vi "Parsing Equations for Linear Optimization.vi"(10 "Variables":string, 11 "Equation":string) -> (0 "error out":errorcluster, 1 "Symbol output":string, 2 "left side":dbl, 3 "Vector":dbl[](array[numeric]), 4 "After symbol":string, 5 "Before symbol":string)   [LabVIEW 2023]
doc: "Parse equation for linear optimization."
uses:
  <vilib>/Utility/error.llb/Trim Whitespace One-Sided.vi
  <vilib>/gmath/NI_Gmath.lvlib
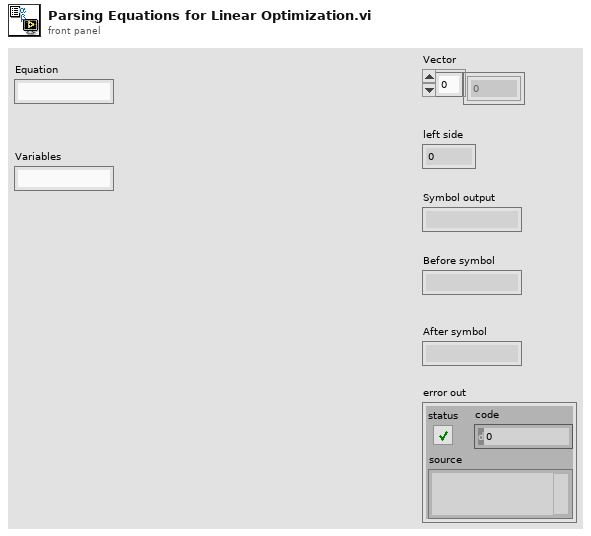
[diagram p1: front panel]
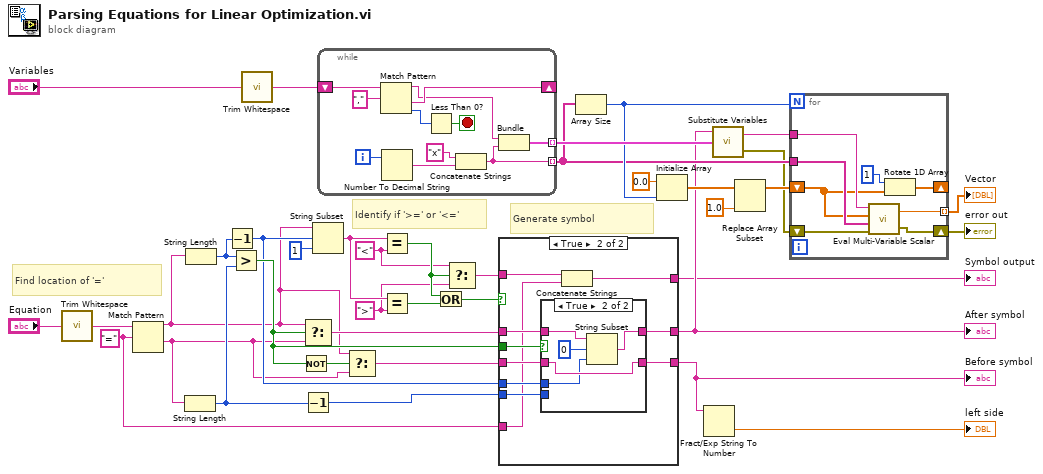
[diagram p0: block diagram]
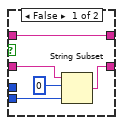
[diagram p3: hidden frame]
diagram:
  w5 = ">" ("y")
  w6 = "<" ("y")
  w9 = "=" ("symbol")
  # "Generate symbol"
  # "Identify if '>=' or '<='"
  # "Find location of '='"
  n1 = call <vilib>:"Trim Whitespace.vi"("string"="Equation") -> ("trimmed string"=w37:string)  [unwired: 1 in]
  n2 = Match Pattern(string=w37, regular expression=w9) -> (before substring=w2:string, after substring=w1:string)  [unwired: 1 in, 2 out]
  n3 = String Length(string=w1) -> (length=w13:i32)
  n4 = String Length(string=w2) -> (length=w15:i32)
  n5 = Decrement(x=w15) -> (x-1=w12:i32)
  n6 = Greater?(x=w15, y=w13) -> (0:w14:bool)
  n7 = call <vilib>:"Trim Whitespace.vi"("string"="Variables") -> ("trimmed string"=w35:string)  [unwired: 1 in]
  n8 = Not(x=w14) -> (.not. x?=w19:bool)
  n9 = Select(t=w2, s=w14, f=w1) -> (s? t:f=w16:string)
  n10 = Decrement(x=w13) -> (x-1=w18:i32)
  n11 = String Subset(string=w2, offset (0)=w12, length (rest)=1 ("length (rest)")) -> (substring=w22:string)
  n12 = while {
    shift-right: [w46] -> _
    shift-left: w35 -> [w45]
    tunnel: [w43] -> w34 mode=indexing
    tunnel: [w40] -> w26 mode=indexing
    i -> [w44]
    stop <- w47 stop-if-true
    n13 = Match Pattern(string=w45, regular expression=",") -> (before substring=w42:string, after substring=w46:string, offset past match=w48:i32)  [unwired: 1 in, 1 out]
    n14 = Number To Decimal String(number=w44) -> (decimal integer string=w41:string)  [unwired: 1 in]
    n15 = Less Than 0?(x=w48) -> (x < 0?=w47:bool)
    n16 = Concatenate Strings("x" ("string"), w41) -> (w40:string)
    n17 = Bundle("trimmed string"=w42, w40) -> (w43:cluster{"trimmed string":string, string})  [unwired: 1 in]
  }
  n18 = Select(t=w2, s=w19, f=w1) -> (s? t:f=w17:string)
  n19 = Equal?(x=w22, y=w6) -> (x = y?=w7:bool)
  n20 = Equal?(x=w22, y=w5) -> (x = y?=w23:bool)
  n21 = Or(x=w7, y=w23) -> (x .or. y?=w21:bool)
  n22 = Select(t=w6, s=w7, f=w5) -> (s? t:f=w4:string)
  n23 = case shown="True" w21 {
    tunnel: w16 -> [w52 w58]
    tunnel: w18 -> [_ w62]
    tunnel: [w52 w57] -> w20
    tunnel: w17 -> [w51 w61]
    tunnel: [w51 w60] -> w11
    tunnel: w14 -> [_ w59]
    tunnel: w12 -> [_ w56]
    tunnel: [w50 w54] -> w8
    tunnel: w9 -> [w50 w53]
    tunnel: w4 -> [_ w55]
    frame False {
    }
    frame True {
      n24 = case shown="True" w59 {
        tunnel: w62 -> [w66 _]
        tunnel: w61 -> [w65 w69]
        tunnel: [w64 w69] -> w60
        tunnel: w58 -> [w63 w71]
        tunnel: [w63 w70] -> w57
        tunnel: w56 -> [_ w68]
        frame False {
          n25 = String Subset(string=w65, offset (0)=0, length (rest)=w66) -> (substring=w64:string)
        }
        frame True {
          n26 = String Subset(string=w71, offset (0)=0, length (rest)=w68) -> (substring=w70:string)
        }
      }
      n27 = Concatenate Strings(w55, w53) -> (w54:string)
    }
  }
  "Before symbol" <- w11
  "Symbol output" <- w8
  "After symbol" <- w20
  n28 = Array Size(array=w26) -> (size(s)=w32:i32)
  n29 = Initialize Array(0.0 ("element"), w32) -> (w30:dbl[])
  n30 = Fract/Exp String To Number(string=w11) -> (number=→"left side":dbl)  [unwired: 3 in, 1 out]
  n31 = call <vilib>:"Substitute Variables.vi"("Substitution Rules"=w34, "original formula"=w20) -> ("error out"=w3:errorcluster, "formula after substitution"=w33:string)  [unwired: 1 in]
  n32 = Replace Array Subset(array=w30, new element=1.0 ("new element/subarray")) -> (w28:dbl[])  [unwired: 1 in]
  n33 = for {
    N: w32 -> [_]
    tunnel: w33 -> [w80]
    tunnel: [w79] -> w27 mode=indexing
    tunnel: w26 -> [w78]
    shift-right: [w76] -> _
    shift-left: w28 -> [w75]
    shift-right: [w74] -> w25
    shift-left: w3 -> [w73]
    n34 = call <vilib>:"Eval Multi-Variable Scalar.vi"("error in (no error)"=w73, "Variables"=w78, "X Values"=w75, "formula"=w80) -> ("error out"=w74:errorcluster, "y value"=w79:dbl)
    n35 = Rotate 1D Array(1:w75, 2:1 ("n")) -> (0:w76:dbl[])
  }
  "Vector" <- w27
  "error out" <- w25
